vi "Trav_cluster_Convert.vi"(4 "Traverse line in":T1 {"Carrier_2 Q (l/min)" format="%#.2f"; "Row Duration (mins)" format="%#.1f"; "Row No" min=0; "Trace Gas Concentration (%)" min=0.0 format="%#_4f"; "Carrier_1 Q (l/min)" format="%#.2f"; "Tunnel Speed" format="%#.2f"; "Start X" format="%#.2f"; "Start Y" format="%#.2f"; "Start Z" format="%#.2f"; "End X" format="%#.2f"; "End Y" format="%#.2f"; "End Z" format="%#.2f"; "Averaging time (min)" min=0.0 format="%#.2f"}, 5 "Channel Values In":string[](array[string]), 6 "Row Number":i32, 7 "Channel names":string[](array[string])) -> (0 "Traverse line Out":T1 {"Carrier_2 Q (l/min)" format="%#.2f"; "Row Duration (mins)" format="%#.1f"; "Row No" min=0; "Trace Gas Concentration (%)" min=0.0 format="%#_4f"; "Carrier_1 Q (l/min)" format="%#.2f"; "Tunnel Speed" format="%#.2f"; "Start X" format="%#.2f"; "Start Y" format="%#.2f"; "Start Z" format="%#.2f"; "End X" format="%#.2f"; "End Y" format="%#.2f"; "End Z" format="%#.2f"; "Averaging time (min)" min=0.0 format="%#.2f"})   [LabVIEW 2015]
uses:
  Traverse_cluster.ctl
  Spacing.ctl
  Controls/Multi_run_mode.ctl
  Globals/Trav_pos_global.vi
panel:
  # "X           Y            Z"
  # "Start"
  # "End"
  # "X           Y            Z"
  # "Start"
  # "End"
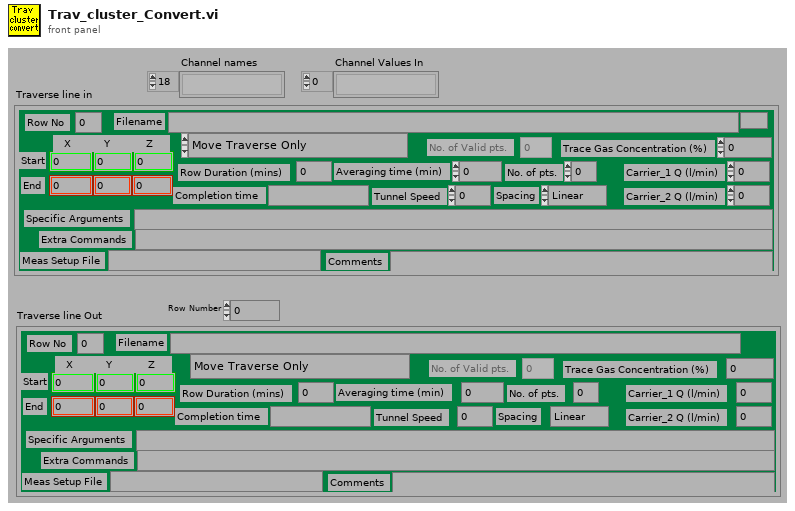
[diagram p1: front panel]
types:
  T1 = typedef "Traverse_cluster.ctl" = cluster{"Start X":sgl, "Start Y":sgl, "Start Z":sgl, "End X":sgl, "End Y":sgl, "End Z":sgl, "No. of pts.":i32, "Spacing":T2, "Filename":path, "Tunnel Speed":dbl, "Averaging time (min)":dbl, "Extra Commands":string, "Carrier_1 Q (l/min)":dbl, "Carrier_2 Q (l/min)":dbl, "Trace Gas Concentration (%)":dbl, "Specific Arguments":string, "Comments":string, "Row No":i32, "Row Type Selector":T3, "Completion time":string, "Row Duration (mins)":dbl, "No. of Valid pts.":i32, "Meas Setup File":string}
  T2 = typedef "Spacing.ctl" = enum16{"Linear", "Log", "Gauss", "Specified", "N/A"}
  T3 = typedef "Multi_run_mode.ctl" = enum16{"Move Traverse Only", "Set Tunnel Speed Only", "Set Source Only", "Set Measurement Conditions", "Single Measurement", "Vertical Profile", "Lateral Profile", "Longitudinal Profile", "Explore Volume", "Multi-Axis Profile", "Auto Calibrate", "Meas Fast FID Bkgnd", "Check Beam Power", "Scanning Valve Measurement", "Run VI Named:", "Set ADAM Ch", "Wait (minutes)", "Send Message", "Synchronize With:", "Fall Back to this Row", "Turn Off Row Repeating", "Blank Row", "Traverse 3D Volume"}
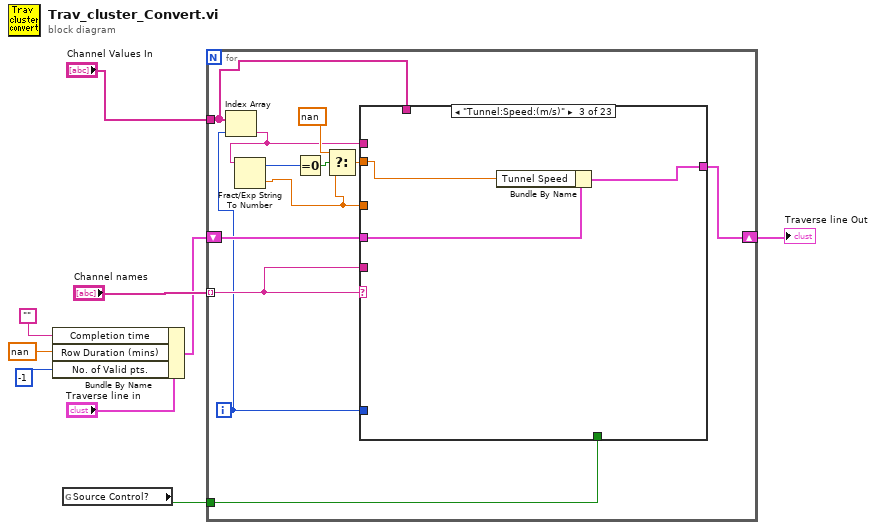
[diagram p0: block diagram]
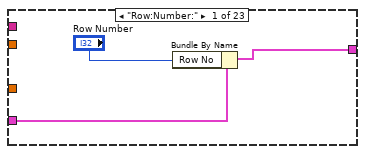
[diagram p2: hidden frame]
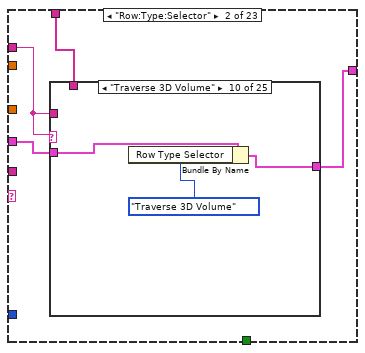
[diagram p3: hidden frame]
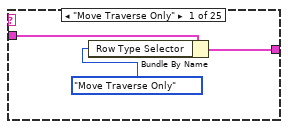
[diagram p4: hidden frame]
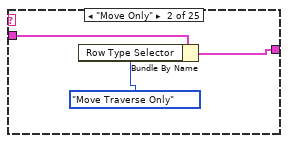
[diagram p5: hidden frame]
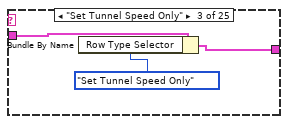
[diagram p6: hidden frame]
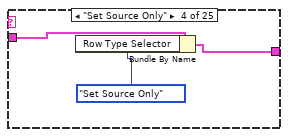
[diagram p7: hidden frame]
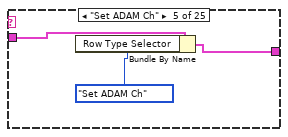
[diagram p8: hidden frame]
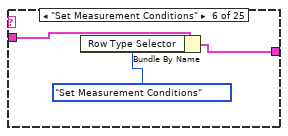
[diagram p9: hidden frame]
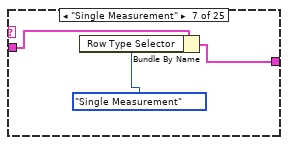
[diagram p10: hidden frame]
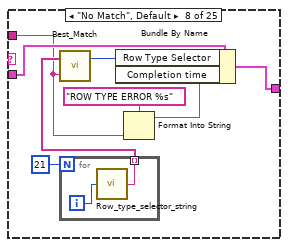
[diagram p11: hidden frame]
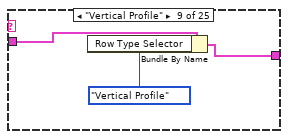
[diagram p12: hidden frame]
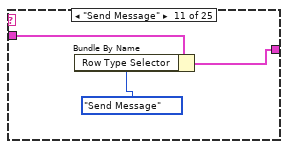
[diagram p13: hidden frame]
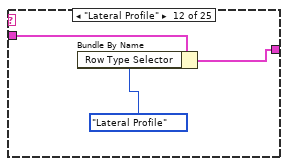
[diagram p14: hidden frame]
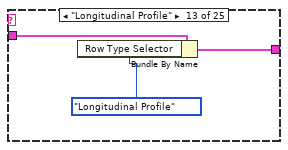
[diagram p15: hidden frame]
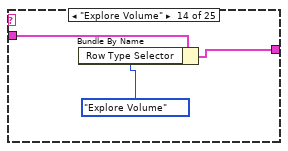
[diagram p16: hidden frame]
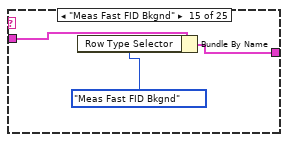
[diagram p17: hidden frame]
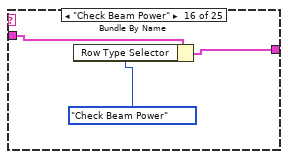
[diagram p18: hidden frame]
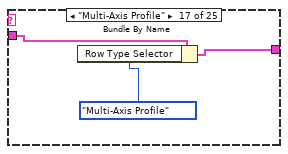
[diagram p19: hidden frame]
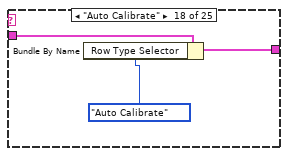
[diagram p20: hidden frame]
diagram:
  n1 = Bundle By Name(cluster="Traverse line in", "Completion time"="", "Row Duration (mins)"=nan ("Bundle Element"), "No. of Valid pts."=-1) -> (w4:T1)
  n2 = global read "Trav_pos_global.vi" "Source Control?"() -> (w9:bool)
  n3 = for {
    tunnel: "Channel names" -> [w14] mode=indexing
    shift-right: [w19] -> w3
    shift-left: w4 -> [w21]
    tunnel: w9 -> [w20]
    tunnel: "Channel Values In" -> [w11]
    i -> [w12]
    n4 = Index Array(array=w11, index=w12) -> (element=w13:string)
    n5 = Fract/Exp String To Number(string=w13) -> (offset past number=w18:i32, number=w10:dbl)  [unwired: 1 in, 2 out]
    n6 = Equal To 0?(x=w18) -> (x = 0?=w17:bool)
    n7 = Select(t=nan ("f"), s=w17, f=w10) -> (s? t:f=w16:dbl)
    n8 = case shown="\"Tunnel:Speed:(m/s)\"" w14 {
      tunnel: w21 -> [w23 w27 w112 w115 w118 w122 w125 w127 w130 w132 w142 w148 w151 w156 w160 w163 w164 w167 w170 w176 w182 w183 w185]
      tunnel: w14 -> [_ _ _ _ _ _ _ _ _ _ _ _ _ _ _ _ _ _ _ _ _ _ w184]
      tunnel: w10 -> [_ _ _ _ _ _ _ _ _ w135 _ w147 _ _ _ _ w166 w169 w172 _ _ _ _]
      tunnel: [w24 w26 w113 w116 w119 w121 w124 w128 w131 w138 w141 w149 w154 w157 w159 w162 w165 w168 w171 w178 w182 w183 w185] -> w19
      tunnel: w13 -> [_ w28 _ _ _ _ _ _ _ _ w140 _ w153 w155 w158 w161 _ _ _ w175 _ _ _]
      tunnel: w20 -> [_ _ _ _ _ _ _ _ _ _ _ _ _ _ _ _ _ _ _ _ _ _ _]
      tunnel: w12 -> [_ _ _ _ _ _ _ _ _ _ _ _ _ _ _ _ _ _ _ _ _ _ _]
      tunnel: w16 -> [_ _ w111 w114 w117 w120 w123 w126 w129 _ _ _ _ _ _ _ _ _ _ _ _ _ _]
      tunnel: w11 -> [_ w25 _ _ _ _ _ _ _ _ _ _ _ _ _ _ _ _ _ w173 _ _ _]
      frame "Row:Number:" {
        n9 = Bundle By Name(cluster=w23, "Row No"="Row Number") -> (w24:T1)
      }
      frame "Row:Type:Selector" {
        n10 = case shown="\"Traverse 3D Volume\"" w28 {
          tunnel: w28 -> [_ _ _ _ _ _ _ w52 _ _ _ _ _ _ _ _ _ _ _ _ _ _ _ _ _]
          tunnel: w27 -> [w31 w33 w36 w39 w42 w45 w48 w54 w61 w64 w67 w71 w73 w77 w79 w82 w85 w89 w91 w94 w97 w100 w103 w106 w109]
          tunnel: [w30 w32 w35 w38 w41 w44 w47 w53 w62 w65 w66 w70 w72 w75 w78 w81 w84 w88 w90 w93 w96 w99 w102 w105 w110] -> w26
          tunnel: w25 -> [_ _ _ _ _ _ _ _ _ _ _ _ _ _ _ _ _ _ _ _ _ _ _ _ _]
          frame "Move Traverse Only" {
            n11 = Bundle By Name(cluster=w31, "Row Type Selector"=Multi_run_mode."Move Traverse Only" ("Mode")) -> (w30:T1)
          }
          frame "Move Only" {
            n12 = Bundle By Name(cluster=w33, "Row Type Selector"=Multi_run_mode."Move Traverse Only" ("Mode")) -> (w32:T1)
          }
          frame "Set Tunnel Speed Only" {
            n13 = Bundle By Name(cluster=w36, "Row Type Selector"=Multi_run_mode."Set Tunnel Speed Only" ("Mode")) -> (w35:T1)
          }
          frame "Set Source Only" {
            n14 = Bundle By Name(cluster=w39, "Row Type Selector"=Multi_run_mode."Set Source Only" ("Mode")) -> (w38:T1)
          }
          frame "Set ADAM Ch" {
            n15 = Bundle By Name(cluster=w42, "Row Type Selector"=Multi_run_mode."Set ADAM Ch" ("Mode")) -> (w41:T1)
          }
          frame "Set Measurement Conditions" {
            n16 = Bundle By Name(cluster=w45, "Row Type Selector"=Multi_run_mode."Set Measurement Conditions" ("Mode")) -> (w44:T1)
          }
          frame "Single Measurement" {
            n17 = Bundle By Name(cluster=w48, "Row Type Selector"=Multi_run_mode."Single Measurement" ("Mode")) -> (w47:T1)
          }
          frame "No Match", Default {
            n18 = for {
              N: 21 -> [_]
              tunnel: [w58] -> w56 mode=indexing
              i -> [w59]
              n19 = call "Row_type_selector_string.vi"("Mode"=w59) -> ("Output string"=w58:string)
            }
            n20 = call "Best_Match.vi"("Input String"=w52, "String Options"=w56) -> ("index of element"=w55:i32)  [unwired: 1 out]
            n21 = Format Into String(format string="ROW TYPE ERROR %s", w52) -> (resulting string=w50:string)  [unwired: 2 in, 1 out]
            n22 = Bundle By Name(cluster=w54, "Row Type Selector"=w55, "Completion time"=w50) -> (w53:T1)
          }
          frame "Vertical Profile" {
            n23 = Bundle By Name(cluster=w61, "Row Type Selector"=Multi_run_mode."Vertical Profile" ("Mode")) -> (w62:T1)
          }
          frame "Traverse 3D Volume" {
            n24 = Bundle By Name(cluster=w64, "Row Type Selector"=Multi_run_mode."Traverse 3D Volume" ("Mode")) -> (w65:T1)
          }
          frame "Send Message" {
            n25 = Bundle By Name(cluster=w67, "Row Type Selector"=Multi_run_mode."Send Message" ("Mode")) -> (w66:T1)
          }
          frame "Lateral Profile" {
            n26 = Bundle By Name(cluster=w71, "Row Type Selector"=Multi_run_mode."Lateral Profile" ("Mode")) -> (w70:T1)
          }
          frame "Longitudinal Profile" {
            n27 = Bundle By Name(cluster=w73, "Row Type Selector"=Multi_run_mode."Longitudinal Profile" ("Mode")) -> (w72:T1)
          }
          frame "Explore Volume" {
            n28 = Bundle By Name(cluster=w77, "Row Type Selector"=Multi_run_mode."Explore Volume" ("Mode")) -> (w75:T1)
          }
          frame "Meas Fast FID Bkgnd" {
            n29 = Bundle By Name(cluster=w79, "Row Type Selector"=Multi_run_mode."Meas Fast FID Bkgnd" ("Mode")) -> (w78:T1)
          }
          frame "Check Beam Power" {
            n30 = Bundle By Name(cluster=w82, "Row Type Selector"=Multi_run_mode."Check Beam Power" ("Mode")) -> (w81:T1)
          }
          frame "Multi-Axis Profile" {
            n31 = Bundle By Name(cluster=w85, "Row Type Selector"=Multi_run_mode."Multi-Axis Profile" ("Mode")) -> (w84:T1)
          }
          frame "Auto Calibrate" {
            n32 = Bundle By Name(cluster=w89, "Row Type Selector"=Multi_run_mode."Auto Calibrate" ("Mode")) -> (w88:T1)
          }
          frame "Scanning Valve Measurement" {
            n33 = Bundle By Name(cluster=w91, "Row Type Selector"=Multi_run_mode."Scanning Valve Measurement" ("Mode")) -> (w90:T1)
          }
          frame "Wait (minutes)" {
            n34 = Bundle By Name(cluster=w94, "Row Type Selector"=Multi_run_mode."Wait (minutes)" ("Mode")) -> (w93:T1)
          }
          frame "Run VI Named:" {
            n35 = Bundle By Name(cluster=w97, "Row Type Selector"=Multi_run_mode."Run VI Named:" ("Mode")) -> (w96:T1)
          }
          frame "Synchronize With:" {
            n36 = Bundle By Name(cluster=w100, "Row Type Selector"=Multi_run_mode."Synchronize With:" ("Mode")) -> (w99:T1)
          }
          frame "Fall Back to this Row" {
            n37 = Bundle By Name(cluster=w103, "Row Type Selector"=Multi_run_mode."Fall Back to this Row" ("Mode")) -> (w102:T1)
          }
          frame "Turn Off Row Repeating" {
            n38 = Bundle By Name(cluster=w106, "Row Type Selector"=Multi_run_mode."Turn Off Row Repeating" ("Mode")) -> (w105:T1)
          }
          frame "" {
            n39 = Bundle By Name(cluster=w109, "Row Type Selector"=Multi_run_mode."Blank Row" ("Mode")) -> (w110:T1)
          }
        }
      }
      frame "Tunnel:Speed:(m/s)" {
        n40 = Bundle By Name(cluster=w112, "Tunnel Speed"=w111) -> (w113:T1)
      }
      frame "Start at:X:(mm)" {
        n41 = Bundle By Name(cluster=w115, "Start X"=w114) -> (w116:T1)
      }
      frame "Start at:Y:(mm)" {
        n42 = Bundle By Name(cluster=w118, "Start Y"=w117) -> (w119:T1)
      }
      frame "Start at:Z:(mm)" {
        n43 = Bundle By Name(cluster=w122, "Start Z"=w120) -> (w121:T1)
      }
      frame "End at:X:(mm)" {
        n44 = Bundle By Name(cluster=w125, "End X"=w123) -> (w124:T1)
      }
      frame "End at:Y:(mm)" {
        n45 = Bundle By Name(cluster=w127, "End Y"=w126) -> (w128:T1)
      }
      frame "End at:Z:(mm)" {
        n46 = Bundle By Name(cluster=w130, "End Z"=w129) -> (w131:T1)
      }
      frame "Number:Of:Points" {
        n47 = Not A Number/Path/Refnum?(number/path/refnum=w135) -> (NaN/Path/Refnum?=w137:bool)
        n48 = To Long Integer(number=w135) -> (32bit integer=w136:i32)
        n49 = Select(t=0, s=w137, f=w136) -> (s? t:f=w133:i32)
        n50 = Bundle By Name(cluster=w132, "No. of pts."=w133) -> (w138:T1)
      }
      frame "Point:Spacing:Method" {
        n51 = case shown="\"Linear\", Default" w140 {
          tunnel: [Spacing."Linear" ("Spacing") Spacing."Log" ("Spacing") Spacing."Gauss" ("Spacing") Spacing."Specified" ("Spacing")] -> w139
          frame "Linear", Default {
          }
          frame "Log" {
          }
          frame "Gauss" {
          }
          frame "Specified" {
          }
        }
        n52 = Bundle By Name(cluster=w142, "Spacing"=w139) -> (w141:T1)
      }
      frame "Averaging:Time:(mins)" {
        n53 = Bundle By Name(cluster=w148, "Averaging time (min)"=w147) -> (w149:T1)
      }
      frame "Filename:HD:Users" {
        n54 = call "Text_without_format.vi"("Input string"=w153) -> ("Output string"=w152:string)
        n55 = String To Path(string=w152) -> (path=w150:path)
        n56 = Bundle By Name(cluster=w151, "Filename"=w150) -> (w154:T1)
      }
      frame "Specific:Arguments:String" {
        n57 = Bundle By Name(cluster=w156, "Specific Arguments"=w155) -> (w157:T1)
      }
      frame "Measurement:Setup:File" {
        n58 = Bundle By Name(cluster=w160, "Meas Setup File"=w158) -> (w159:T1)
      }
      frame "Extra:Commands:String" {
        n59 = Bundle By Name(cluster=w163, "Extra Commands"=w161) -> (w162:T1)
      }
      frame "Carrier_1:Q:(l/min)" {
        n60 = Bundle By Name(cluster=w164, "Carrier_1 Q (l/min)"=w166) -> (w165:T1)
      }
      frame "Carrier_2:Q:(l/min)" {
        n61 = Bundle By Name(cluster=w167, "Carrier_2 Q (l/min)"=w169) -> (w168:T1)
      }
      frame "Trace Gas:Concentration:(%)" {
        n62 = Bundle By Name(cluster=w170, "Trace Gas Concentration (%)"=w172) -> (w171:T1)
      }
      frame "Comments::" {
        n63 = Unbundle By Name(w176) -> ("Row Type Selector"=w177:T3)
        n64 = case shown="\"Blank Row\"" w177 {
          tunnel: [w179 w180] -> w174
          tunnel: w175 -> [w179 _]
          tunnel: w173 -> [_ w181]
          frame "Set ADAM Ch", Default {
          }
          frame "Blank Row" {
            n65 = Concatenate Strings(w181) -> (w180:string)
          }
        }
        n66 = Bundle By Name(cluster=w176, "Comments"=w174) -> (w178:T1)
      }
      frame "Row:Completion:Time" {
      }
      frame "Time:Taken in:Row (mins)" {
      }
      frame "No match", Default {
        n67 = call "Was_string_matched.vi"("Variable name"=w184) -> ()  [unwired: 2 in]
      }
    }
  }
  "Traverse line Out" <- w3
